vi "Mono_ReadGratingJose.vi"(8 "error in (no error) 2":errorcluster, 11 "CmdLib In":refnum<k24>) -> (0 "error out 2":errorcluster, 2 "Current Grating":string, 3 "CmdLib Out":refnum<k24>)   [LabVIEW 2017]
uses:
  C:/Users/Admin/Desktop/Sensitive EQE Stuff/S-EQE (YJ)/Mono vi (YJ)/Cornerstone.dll
  Cornerstone.dll
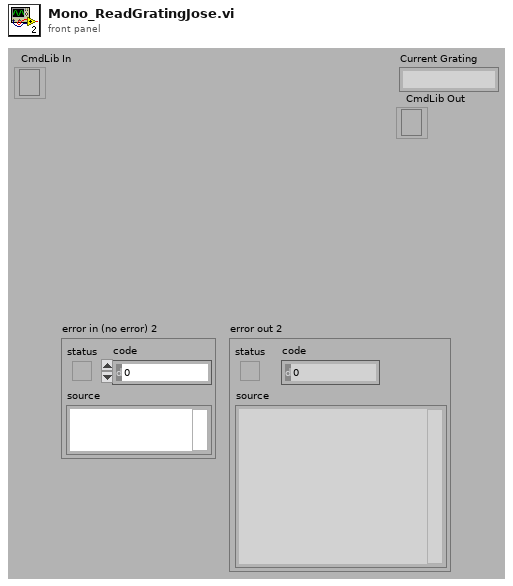
[diagram p1: front panel]
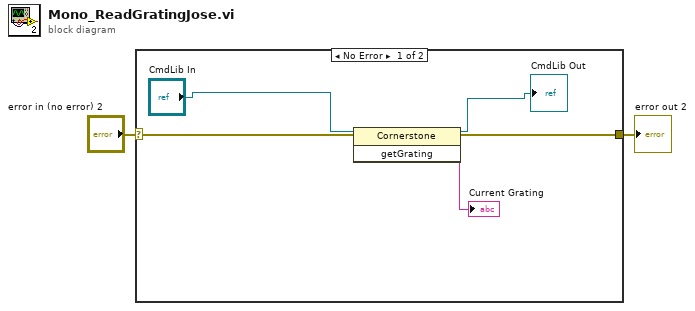
[diagram p0: block diagram]
diagram:
  n1 = case shown="No Error" "error in (no error) 2" {
    selector: "error in (no error) 2" -> [w7 w8]
    tunnel: [w6 w8] -> w1
    frame No Error {
      n2 = invoke class="Cornerstone" method="getGrating"(reference="CmdLib In", error in=w7) -> (reference out=→"CmdLib Out":refnum<k24>, error out=w6:errorcluster, "getGrating"=→"Current Grating":string)  [unwired: 1 in]
    }
    frame Error {
    }
  }
  "error out 2" <- w1
